vi "Get Analog and Digital Values.vi"(8 "error in (no error)":errorcluster, 11 "Output Sequencer in":refnum<class "Output Sequencer.lvclass">) -> (0 "error out":errorcluster, 1 "Digital Values to Write":bool[](array[boolean]), 2 "Analog Values to Write":dbl[](array[numeric]), 3 "Output Sequencer out":refnum<class "Output Sequencer.lvclass">)   [LabVIEW 2020, in "Output Sequencer.lvlib" / "Output Sequencer.lvclass"]
uses:
  Output Sequencer.lvclass
  Output Sequencer.lvclass/Output Sequencer.ctl
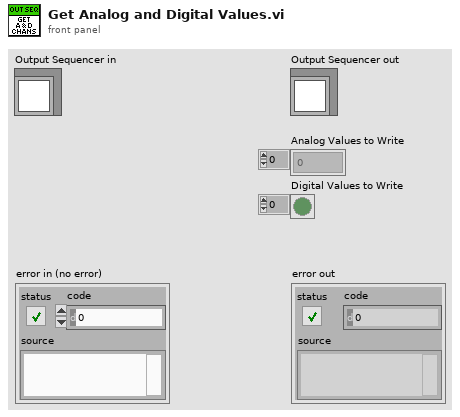
[diagram p1: front panel]
types:
  T1 = typedef "Output Sequencer.lvlib/Output Sequencer.lvclass/Compiled Step.ctl" = cluster{"Precondition":T2, "Duration":dbl, "Mode":string, "Delay Between Values":dbl, "Analog Values":T2[], "Digital Values":T2[], "Postcondition":T2, "On True":string, "On False":string}
  T2 = typedef "Output Sequencer.lvlib/Output Sequencer.lvclass/Expression Data.ctl" = cluster{"Empty?":bool, "Expression":refnum<class "mupExpr.lvclass">, "Variable Names":string[]}
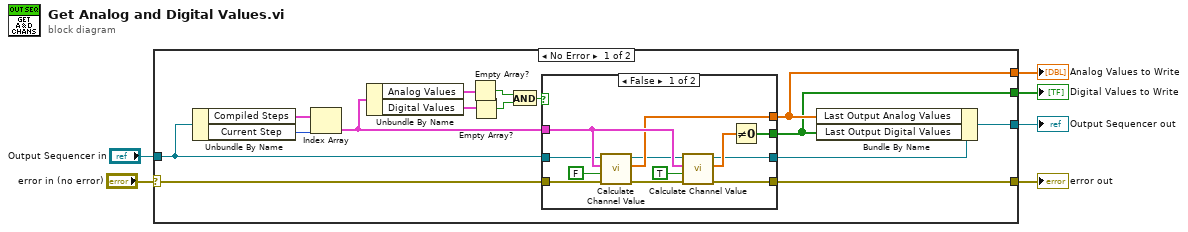
[diagram p0: block diagram]
diagram:
  n1 = case shown="No Error" "error in (no error)" {
    selector: "error in (no error)" -> [w7 w37]
    tunnel: [w15 w36] -> w6
    tunnel: [w14 _] -> w5
    tunnel: [w13 _] -> w4
    tunnel: "Output Sequencer in" -> [w12 w36]
    tunnel: [w10 w37] -> w2
    frame No Error {
      n2 = Unbundle By Name(w12) -> ("Compiled Steps"=w8:T1[], "Current Step"=w9:i32)
      n3 = Index Array(array=w8, index=w9) -> (element=w11:T1)
      n4 = Unbundle By Name(w11) -> ("Analog Values"=w21:T2[], "Digital Values"=w20:T2[])
      n5 = Empty Array?(array=w21) -> (empty?=w19:bool)
      n6 = Empty Array?(array=w20) -> (empty?=w18:bool)
      n7 = And(x=w19, y=w18) -> (x .and. y?=w17:bool)
      n8 = case shown="False" w17 {
        tunnel: w11 -> [w30 _]
        tunnel: [w29 _] -> w14
        tunnel: [w31 _] -> w13
        tunnel: [w25 w35] -> w16
        tunnel: w12 -> [w27 w35]
        tunnel: w7 -> [w24 w34]
        tunnel: [w22 w34] -> w10
        frame False {
          n9 = call "Calculate Channel Value.vi"("error in (no error)"=w24, "Digital"=FALSE, "Step Settings"=w30, "Output Sequencer in"=w27) -> ("error out"=w23:errorcluster, "Values to Write"=w29:dbl[], "Output Sequencer out"=w26:refnum<class "Output Sequencer.lvclass">)  [unwired: 5 in]
          n10 = call "Calculate Channel Value.vi"("error in (no error)"=w23, "Digital"=TRUE, "Step Settings"=w30, "Output Sequencer in"=w26) -> ("error out"=w22:errorcluster, "Values to Write"=w28:dbl[], "Output Sequencer out"=w25:refnum<class "Output Sequencer.lvclass">)  [unwired: 5 in]
          n11 = Not Equal To 0?(x=w28) -> (x != 0?=w31:bool[])
        }
        frame True {
        }
      }
      n12 = Bundle By Name(cluster=w16, "Last Output Analog Values"=w14, "Last Output Digital Values"=w13) -> (w15:refnum<class "Output Sequencer.lvclass">)
    }
    frame Error {
    }
  }
  "Analog Values to Write" <- w5
  "Digital Values to Write" <- w4
  "Output Sequencer out" <- w6
  "error out" <- w2
